vi "CoriolisCompensate.vi"(10 "Coriolis  Data":T1={"Cluster"={"Density_g_L"=1000.0, "FLow(ul/min)"=1000.0, "Temperature(C)"=20.0}, "current time"=timestamp(0 s since 1904-01-01)}, 11 "Cluster":T2={"A1"=6.4106, "A2"=0.998, "B"=-0.3465, "C1"=-0.016457, "C2"=3.3383e-05}) -> (3 "Compensated Density":dbl=1014.4066000000001)   [LabVIEW 2023]
panel:
  # "Rho20=A1+A2*Rhomeas+B*Tmeas+C1*Qmeas+C2*Qmeas^2"
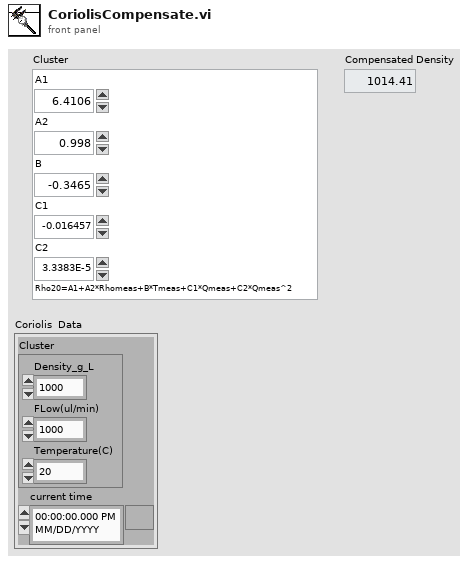
[diagram p1: front panel]
types:
  T1 = cluster{"Cluster":cluster{"Density_g_L":sgl, "FLow(ul/min)":sgl, "Temperature(C)":sgl}, "current time":timestamp}
  T2 = cluster{"A1":dbl, "A2":dbl, "B":dbl, "C1":dbl, "C2":dbl}
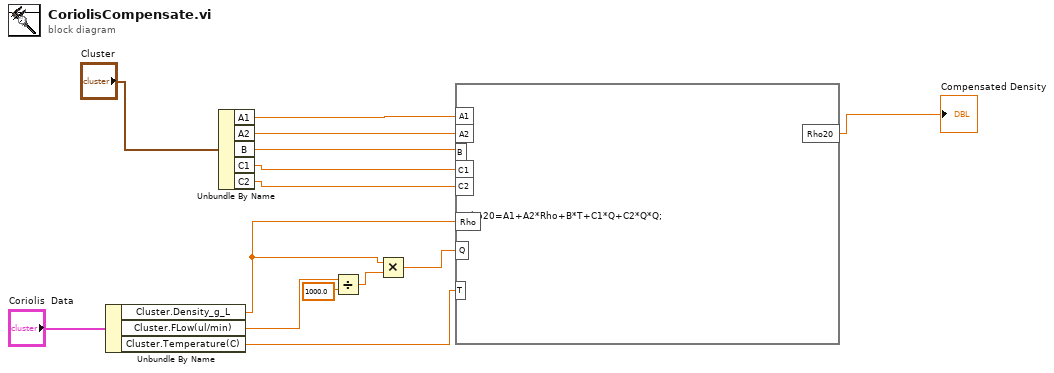
[diagram p0: block diagram]
diagram:
  n1 = Unbundle By Name("Coriolis  Data") -> ("Cluster.Density_g_L"=w5:sgl, "Cluster.FLow(ul/min)"=w2:sgl, "Cluster.Temperature(C)"=w7:sgl)
  n2 = Unbundle By Name("Cluster") -> ("A1"=w13:dbl, "A2"=w12:dbl, "B"=w11:dbl, "C1"=w10:dbl, "C2"=w9:dbl)
  n3 = Divide(x=w2, y=1000.0) -> (x/y=w1:dbl)
  n4 = Multiply(x=w5, y=w1) -> (x*y=w4:dbl)
  n5 = formula code="Rho20=A1+A2*Rho+B*T+C1*Q+C2*Q*Q;"("A1"=w13, "A2"=w12, "B"=w11, "C1"=w10, "C2"=w9, "Rho"=w5, "Q"=w4, "T"=w7) -> ("Rho20"=→"Compensated Density":dbl)
